vi "uTTA_FlushSerialBuffer.vi"(4 "error in (no error)":errorcluster, 7 "VISA Refnum in":refnum<visa-resource-name>) -> (0 "error out":errorcluster, 3 "VISA Refnum out":refnum<visa-resource-name>)   [LabVIEW 2021]
uses:
  uTTA_GV_Serial_Monitor.vi
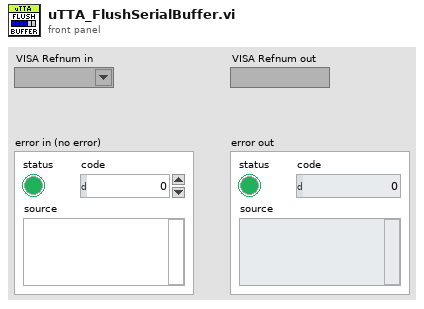
[diagram p1: front panel]
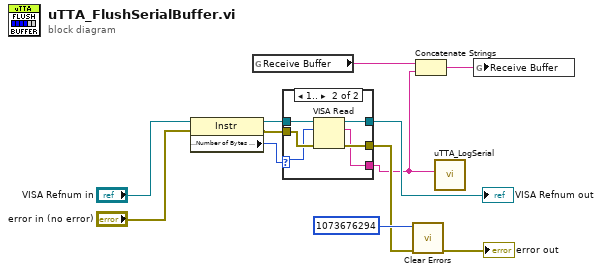
[diagram p0: block diagram]
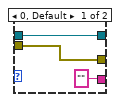
[diagram p2: hidden frame]
diagram:
  n1 = property class="Instr"(reference="VISA Refnum in", error in="error in (no error)") -> (reference out=w7:refnum<visa-resource-name>, error out=w8:errorcluster, "Serial Settings:Number of Bytes at Serial Port"=w9:u32)
  n2 = global read "uTTA_GV_Serial_Monitor.vi" "Receive Buffer"() -> (w3:string)
  n3 = case shown="1.." w9 {
    selector: w9 -> [_ w19]
    tunnel: w7 -> [w15 w21]
    tunnel: w8 -> [w14 w20]
    tunnel: [w15 w18] -> w12
    tunnel: [w14 w17] -> w5
    tunnel: ["" ("read buffer") w16] -> w2
    frame 0, Default {
    }
    frame 1.. {
      n4 = VISA Read(VISA resource name=w21, byte count=w19, error in (no error)=w20) -> (VISA resource name out=w18:refnum<visa-resource-name>, read buffer=w16:string, error out=w17:errorcluster)  [unwired: 1 out]
    }
  }
  "VISA Refnum out" <- w12
  n5 = call <vilib>:"Clear Errors.vi"("error in (no error)"=w5, "specific error code to clear (0: all)"=1073676294) -> ("error out"=→"error out":errorcluster)  [unwired: 4 in, 1 out]
  n6 = Concatenate Strings(w3, w2) -> (w1:string)
  n7 = call "uTTA_LogSerial.vi"("Data_Sent"=w2) -> ()  [unwired: 6 in, 1 out]
  n8 = global write "uTTA_GV_Serial_Monitor.vi" "Receive Buffer"(w1) -> ()
